vi "Read Assert Factory.vi"(8 "error in (no error)":errorcluster) -> (0 "error out":errorcluster, 3 "Assert Factory":refnum<class "Assert Factory.lvclass">)   [LabVIEW 2009, in "Caraya.lvlib" / "Assert Factory Global.lvclass"]
uses:
  Assert Factory Global.lvclass
  Assert Factory/Assert Factory.lvclass
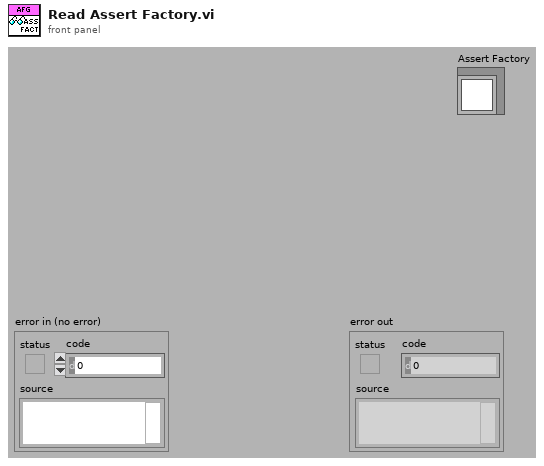
[diagram p1: front panel]
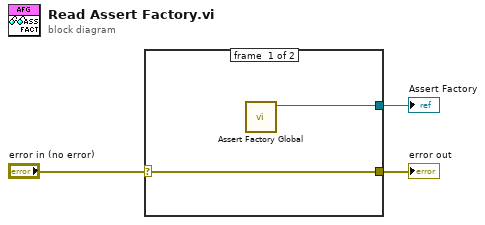
[diagram p0: block diagram]
diagram:
  n1 = case shown="No Error" "error in (no error)" {
    selector: "error in (no error)" -> [w4 w6]
    tunnel: [w5 _] -> w3
    tunnel: [w4 w6] -> w1
    frame #0 {
      n2 = call "Assert Factory Global.vi"() -> ("Assert Factory out"=w5:refnum<class "Assert Factory.lvclass">)  [unwired: 9 in, 2 out]
    }
    frame #1 {
    }
  }
  "Assert Factory" <- w3
  "error out" <- w1
